vi "Get Gyro Angle.vi"(1 "refnum name":string="My Gyro RefNum") -> (0 "Angle":dbl)   [LabVIEW 2016]
doc: "Get a normalized (0 to 360) gyro angle."
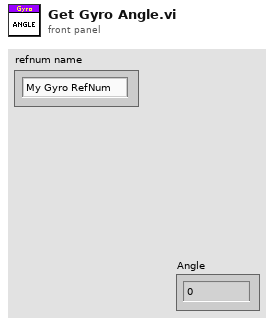
[diagram p1: front panel]
types:
  T1 = typedef "WPI_GyroDevRef.ctl" = cluster{"DevStatus":errorcluster, "Analog Channel":T2, "Offset":dbl, "Gain (VoltsPerDegree/Second)":dbl, "Gyro Type":enum16{"Analog", "XRS450"}, "Handle":i32, "SPI Bus":T3, "Device Found":bool, "Sample Rate":dbl, "Calibrate On Open":bool}
  T2 = typedef "FPGA_AIChannel.ctl" = enum8{"AI 0", "AI 1", "AI 2", "AI 3", "AI MXP 0", "AI MXP 1", "AI MXP 2", "AI MXP 3", "Invalid"}
  T3 = typedef "spi_bus.ctl" = enum16{"SPI On-Board, CS0", "SPI On-Board, CS1", "SPI On-Board, CS2", "SPI On-Board, CS3", "SPI MXP", "Invalid"}
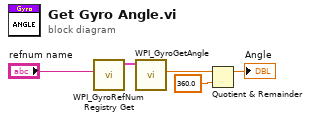
[diagram p0: block diagram]
diagram:
  n1 = call <vilib>:"WPI_GyroRefNum Registry Get.vi"("refnum name"="refnum name") -> ("GyroDevRef"=w5:T1)  [unwired: 9 in, 1 out]
  n2 = call <vilib>:"WPI_GyroGetAngle.vi"("GyroDevRef"=w5) -> ("Angle"=w1:dbl)  [unwired: 7 in, 3 out]
  n3 = Quotient & Remainder(x=w1, y=360.0) -> (x-y*floor(x/y)=→"Angle":dbl)  [unwired: 1 out]
